vi "TEST - Random Number - Within Range.vi"(8 "error in (no error)":errorcluster) -> (0 "error out":errorcluster, 2 "pass":bool)   [LabVIEW 2009]
uses:
  <vilib>/Analysis/NI_AALBase.lvlib
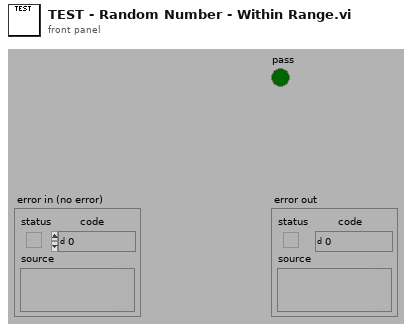
[diagram p1: front panel]
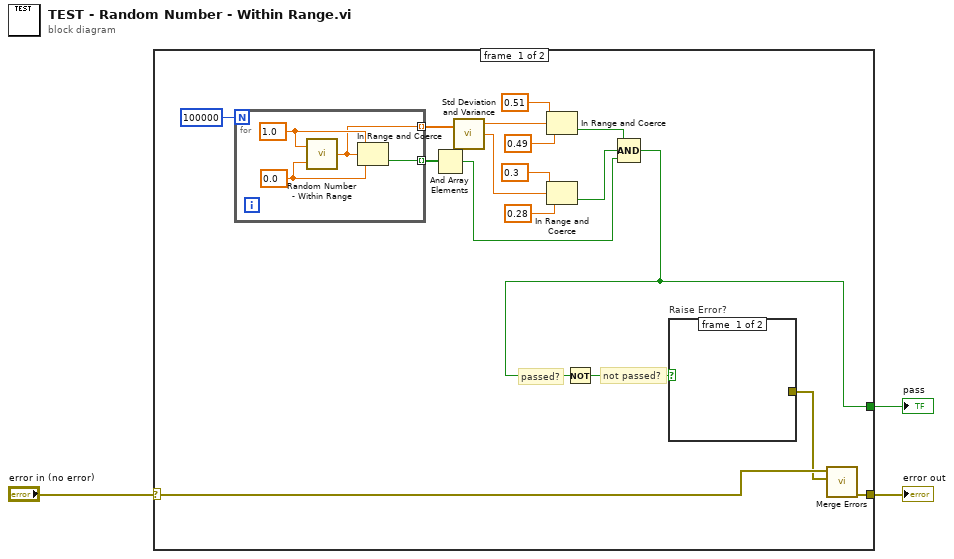
[diagram p0: block diagram]
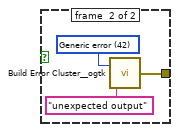
[diagram p2: hidden frame]
diagram:
  n1 = case shown="No Error" "error in (no error)" {
    selector: "error in (no error)" -> [w20 w28]
    tunnel: [w4 _] -> w3
    tunnel: [w19 w28] -> w1
    frame #0 {
      # "not passed?"
      # "passed?"
      n2 = for {
        N: 100000 -> [_]
        tunnel: [w22] -> w15 mode=indexing
        tunnel: [w21] -> w14 mode=indexing
        w23 = 0.0 ("Low (0.00)")
        w24 = 1.0 ("High (1.00)")
        n3 = call "Random Number - Within Range.vi"("High (1.00)"=w24, "Low (0.00)"=w23) -> ("Random #"=w21:dbl)  [unwired: 3 in]
        n4 = In Range and Coerce(upper limit=w24, x=w21, lower limit=w23) -> (In Range?=w22:bool)  [unwired: 1 out]
      }
      n5 = And Array Elements(Boolean array=w15) -> (logical AND=w5:bool)
      n6 = call <vilib>:"Std Deviation and Variance.vi"("X"=w14) -> ("mean"=w13:dbl, "standard deviation"=w7:dbl)  [unwired: 1 in, 1 out]
      n7 = In Range and Coerce(upper limit=0.51, x=w13, lower limit=0.49 ("upper limit")) -> (In Range?=w10:bool)  [unwired: 1 out]
      n8 = In Range and Coerce(upper limit=0.3, x=w7, lower limit=0.28 ("upper limit")) -> (In Range?=w6:bool)  [unwired: 1 out]
      n9 = Compound Arithmetic op=AND(w10, w6, w5) -> (w4:bool)
      n10 = Not(x=w4) -> (.not. x?=w17:bool)
      n11 = case "Raise Error?" shown="True" w17 {
        tunnel: [_ w25] -> w18
        frame #0 {
        }
        frame #1 {
          w26 = 42 items=["No error", "Argument error", "Memory is full", "Out of zone", "End of file", "File already open", "Generic file I/O error", "File not found", "File permission error", "Disk is full", "Duplicate path", "Too many files open", "System feature not enabled", "Resource file not found", "Cannot add resource", "Resource not found", "Image not found", "Image memory error", "Pen does not exist", "Config type invalid", "Config token not found", "Config parse error", "Config memory error", "Bad external code format", "Bad external code offset", "External code not present", "Null window", "Destroy window error", "Null menu", "Print aborted", "Bad print record", "Print driver error", "Windows error during printing", "Memory error during printing", "Print dialog error", "Generic print error", "Invalid device refnum", "Device not found", "Device parameter error", "Device unit error", "Cannot open device", "Device call aborted", "Generic error", "Cancelled by user", "Object ID too low", "Object ID too high", "Object not in heap", "Unknown heap", "Unknown object (invalid DefProc)", "Unknown object (DefProc not in table)", "Message out of range", "Invalid (null) method", "Unknown message", "Manager call not supported", "Bad address", "Network operation in progress", "Network operation timed out", "Connection is busy", "Network attribute not supported", "Network error", "Address in use", "System out of memory", "Connection aborted", "Connection refused", "Not connected", "Already connected", "Connection closed", "Initialization error (interapplication manager)", "Bad occurrence", "Wait on unbound occurrence handler", "Occurrence queue overflow", "Datalog type conflict", "Unused", "Unrecognized type (interapplication manager)", "Memory corrupt", "Failed to make temporary DLL", "Old CIN version", "Drag socket not found", "Failed to load drop-object", "Failed to register OLE object", "Failed to release OLE object", "Format specifier type mismatch", "Unknown format specifier", "Too few format specifiers", "Too many format specifiers", "Scan failed", "Newer CIN version", "Error converting to variant", "Runtime menu error", "Password tampered", "Variant attribute not found", "Incompatible variant data type", "Event data is not available", "Event Store is not present", "Occurrence is not found", "Event Queue is not created", "Event info is not available", "Refnum passed is NULL", "Error retrieving Class GUID", "Error retrieving CoClass GUID", "Error retrieving TypeLib GUID.", "Bad built application magic bytes.", "Specific driver is different from the specific driver associated with the Logical Name.", "There is no session opened to the class driver.", "Max Error", "MAX - Error with config objects", "MAX - Error loading configuration", "MAX - Group not supported"]
          n12 = call <userlib>:"Build Error Cluster__ogtk.vi"("String to Prepend to source (\"\")"="unexpected output" ("String to Prepend to source (\"\")"), "code"=w26) -> ("error out"=w25:errorcluster)
        }
      }
      n13 = call <vilib>:"Merge Errors.vi"("error in 2 (no error)"=w18, "error in 1 (no error)"=w20) -> ("error out"=w19:errorcluster)  [unwired: 5 in]
    }
    frame #1 {
    }
  }
  "pass" <- w3
  "error out" <- w1
